vi "ReportHead1.vi"(8 "error in (no error)":errorcluster caption="错误输入（无错误）", 11 "产品状态":string) -> (0 "error out":errorcluster caption="错误输出", 3 "report out":refnum<class "NI_report.lvclass"> caption="报表输出")   [LabVIEW 2020]
uses:
  <vilib>/Utility/NIReport.llb/NI_report.lvclass
  <vilib>/addons/_office/_exclsub.llb/font.ctl
  <vilib>/Utility/NIReport.llb/Report Type.ctl
  Database/Global1.vi
  <vilib>/addons/_office/NI_ReportGenerationToolkit.lvlib
  <vilib>/Utility/NIReport.llb/NI_ReportGenerationCore.lvlib
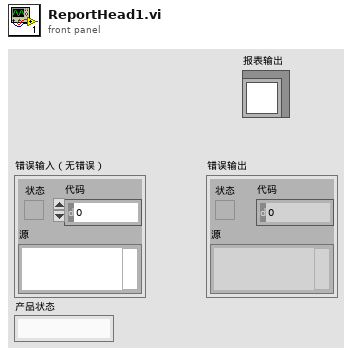
[diagram p1: front panel]
types:
  T1 = typedef "NI_ReportGenerationCore.lvlib/Report Type.ctl" = enum16{"HTML", "Word", "Excel"}
  T2 = enum16{"maximized", "minimized", "normal", "no change"}
  T3 = cluster{"操作者编号":string, "操作者姓名":string, "操作者权限":string, "联机状态":string, "产品型号":string, "产品状态":string}
  T4 = cluster{"top":dbl, "left":dbl, "right":dbl, "bottom":dbl}
  T5 = cluster{"Charset (-1)":i16, "Weight (-1)":i16, "Name":string, "Size":string}
  T6 = cluster{"Italic":enum16{"Italic Unchanged", "Italic On", "Italic Off"}, "Strike Through":enum16{"Strike Through Unchanged", "Strike Through On", "Strike Through Off"}, "Underline":enum16{"Underline Unchanged", "Underline On", "Underline Off"}, "Bold":enum16{"Bold Unchanged", "Bold On", "Bold Off"}}
  T7 = typedef "NI_ReportGenerationToolkit.lvlib/font.ctl" = cluster{"font name":string, "font size":dbl, "bold":u16, "italic":u16, "underline":u16, "strike through":u16, "font color":u32}
  T8 = cluster{"用户编号":string, "用户名":string, "用户密码(密文)":string, "用户权限":string}
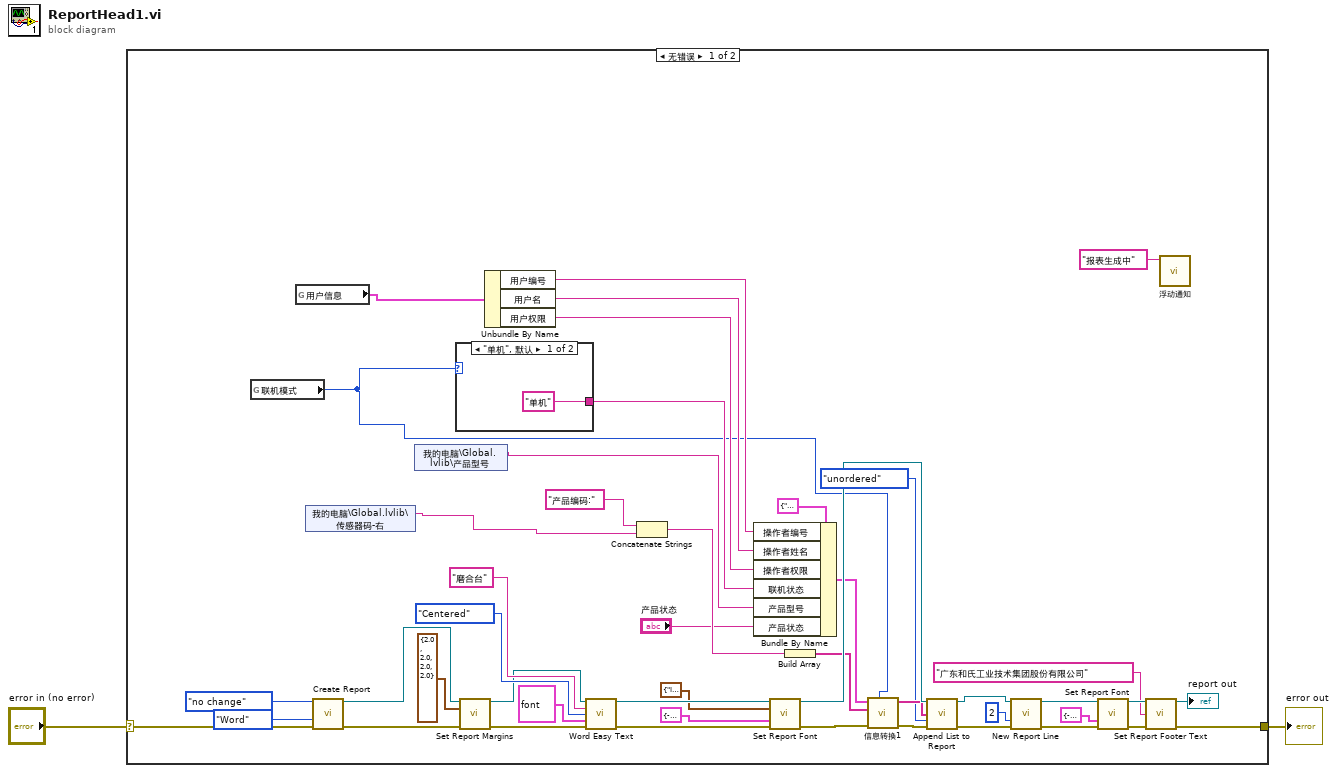
[diagram p0: block diagram]
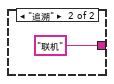
[diagram p2: hidden frame]
diagram:
  n1 = case shown="无错误" "error in (no error)" {
    selector: "error in (no error)" -> [w25 w51]
    tunnel: [w21 w51] -> w1
    frame No Error {
      n2 = global read "Global1.vi" "联机模式"() -> (w4:enum16{"单机", "追溯"})
      n3 = global read "Global1.vi" "用户信息"() -> (w6:T8)
      n4 = shared-variable "我的电脑\\Global.lvlib\\传感器码-右"() -> (w3:string)  [unwired: 1 in, 1 out]
      n5 = call <vilib>:"Create Report.vi"("window state (normal)"=T2."no change", "report type"=Report_Type."Word", "error in (no error)"=w25) -> ("report out"=w38:refnum<class "NI_report.lvclass">, "error out"=w35:errorcluster)  [unwired: 11 in]
      n6 = shared-variable "我的电脑\\Global.lvlib\\产品型号"() -> (w5:string)  [unwired: 1 in, 1 out]
      n7 = case shown="\"单机\", 默认" w4 {
        tunnel: ["单机" "联机"] -> w19
        frame "单机", Default {
        }
        frame "追溯" {
        }
      }
      n8 = call-dynamic "Set Report Margins.vi"("report in"=w38, "margins (1.00)"=T4 {"top"=2.0, "left"=2.0, "right"=2.0, "bottom"=2.0}, "error in (no error)"=w35) -> ("report out"=w37:refnum<class "NI_report.lvclass">, "error out"=w36:errorcluster)  [unwired: 10 in, 1 out]
      n9 = Unbundle By Name(w6) -> ("用户编号"=w9:string, "用户名"=w8:string, "用户权限"=w7:string)
      n10 = call <vilib>:"Word Easy Text.vi"("report in"=w37, "text"="磨合台", "alignment (left)"=enum16{"Left", "Centered", "Right", "Justify"}."Centered", "font"=T7 {"font name"="楷体", "font size"=26.0, "bold"=1, "italic"=2, "underline"=2, "strike through"=2, "font color"=16777228}, "error in (no error)"=w36) -> ("report out"=w46:refnum<class "NI_report.lvclass">, "error out"=w45:errorcluster)  [unwired: 8 in, 1 out]
      n11 = Concatenate Strings("产品编码:", w3) -> (w15:string)
      n12 = Bundle By Name(cluster=T3 {"操作者编号"="001", "操作者姓名"="Administrator", "操作者权限"="系统管理员", "联机状态"="单机", "产品型号"="SL7202", "产品状态"=""} ("测试信息"), "操作者编号"=w9, "操作者姓名"=w8, "操作者权限"=w7, "联机状态"=w19, "产品型号"=w5, "产品状态"="产品状态") -> (w17:T3)
      n13 = call-dynamic "Set Report Font.vi"("report in"=w46, "text options"=T6 {"Italic"=enum."Italic Off", "Strike Through"=enum."Strike Through Unchanged", "Underline"=enum."Underline Off", "Bold"=enum."Bold Off"}, "font settings"=T5 {"Charset (-1)"=-1, "Weight (-1)"=-1, "Name"="微软雅黑 Light", "Size"="12 "}, "error in (no error)"=w45) -> ("report out"=w33:refnum<class "NI_report.lvclass">, "error out"=w24:errorcluster)  [unwired: 9 in, 1 out]
      n14 = Build Array(w15) -> (w14:string[])
      n15 = call "信息转换1.vi"("联机模式"=w4, "错误输入（无错误）"=w24, "追溯码"=w14, "测试信息"=w17) -> ("错误输出"=w23:errorcluster, "信息输出"=w26:string[])  [unwired: 6 in]
      n16 = call-dynamic "Append List to Report.vi"("report in"=w33, "list elements"=w26, "list type (ordered)"=enum16{"unordered", "ordered"}."unordered", "error in (no error)"=w23) -> ("report out"=w28:refnum<class "NI_report.lvclass">, "error out"=w27:errorcluster)  [unwired: 8 in, 2 out]
      n17 = call-dynamic "New Report Line.vi"("report in"=w28, "number of lines (1)"=2, "error in (no error)"=w27) -> ("report out"=w31:refnum<class "NI_report.lvclass">, "error out"=w32:errorcluster)  [unwired: 11 in]
      n18 = call-dynamic "Set Report Font.vi"("report in"=w31, "font settings"=T5 {"Charset (-1)"=-1, "Weight (-1)"=-1, "Name"="楷体", "Size"="9 "}, "error in (no error)"=w32) -> ("report out"=w42:refnum<class "NI_report.lvclass">, "error out"=w41:errorcluster)  [unwired: 10 in, 1 out]
      n19 = call-dynamic "Set Report Footer Text.vi"("report in"=w42, "center footer text"="广东和氏工业技术集团股份有限公司", "error in (no error)"=w41) -> ("report out"=→"report out":refnum<class "NI_report.lvclass">, "error out"=w21:errorcluster)  [unwired: 11 in]
      n20 = call "浮动通知.vi"("通知内容"="报表生成中" ("Status")) -> ()  [unwired: 11 in]
    }
    frame Error {
    }
  }
  "error out" <- w1
